vi "Create from U32.vi"(11 "address U32":u32) -> (3 "address out":refnum<class "IPv4 Network Address.lvclass">)   [LabVIEW 2020, in "NI_WFCN.lvlib" / "IPv4 Network Address.lvclass"]
doc: "Construct an IPv4 Network Address object fom the specified native-byte-order U32 address."
uses:
  <vilib>/net/WFCN/Addressing/IPv4 Network Address/IPv4 Network Address.lvclass
  <vilib>/net/WFCN/Addressing/IPv4 Network Address/IPv4 Network Address.lvclass/IPv4 Network Address.ctl
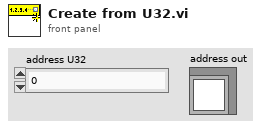
[diagram p1: front panel]
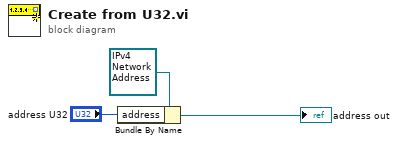
[diagram p0: block diagram]
diagram:
  n1 = Bundle By Name(cluster=refnum<class "IPv4 Network Address.lvclass"> refnum ("IPv4 Network Address in"), "address"="address U32") -> (→"address out":refnum<class "IPv4 Network Address.lvclass">)
